vi "Create quad.vi"(1 "V3":sgl[](array[numeric]), 2 "V2":sgl[](array[numeric]), 3 "V1":sgl[](array[numeric]), 4 "V0":sgl[](array[numeric])) -> (0 "Quad":T1)   [LabVIEW 2014]
uses:
  Typedefs/Quad.ctl
  Dot product.vi
panel:
  # "PN 17/01/2015"
  # "Vertices"
  # "Edges"
  # "Unit normal"
  # "Edge unit normals"
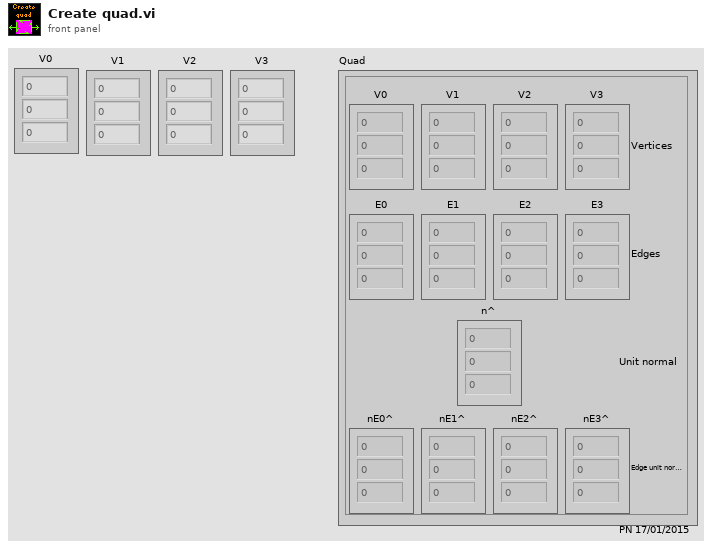
[diagram p1: front panel]
types:
  T1 = typedef "Quad.ctl" = cluster{"V0":sgl[], "V1":sgl[], "V2":sgl[], "V3":sgl[], "E0":sgl[], "E1":sgl[], "E2":sgl[], "E3":sgl[], "n^":sgl[], "nE0^":sgl[], "nE1^":sgl[], "nE2^":sgl[], "nE3^":sgl[]}
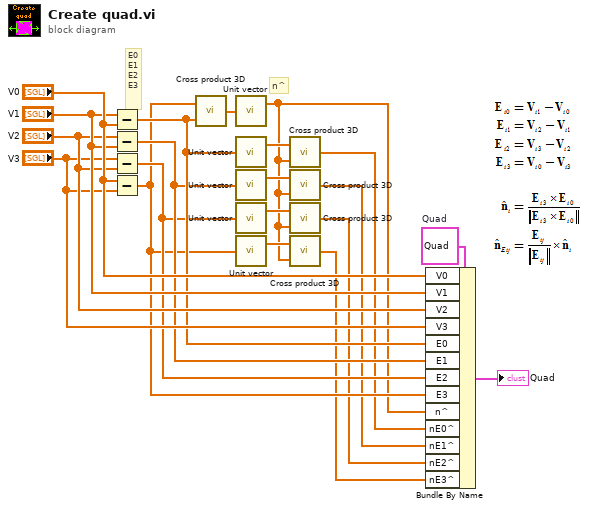
[diagram p0: block diagram]
diagram:
  w19 = T1 {"V0"=[], "V1"=[], "V2"=[], "V3"=[], "E0"=[], "E1"=[], "E2"=[], "E3"=[], "n^"=[], "nE0^"=[], "nE1^"=[], "nE2^"=[], "nE3^"=[]}  # Quad
  # "n^"
  # "E0\nE1\nE2\nE3"
  n1 = Subtract(x="V1", y="V0") -> (x-y=w10:sgl[])
  n2 = Subtract(x="V2", y="V1") -> (x-y=w9:sgl[])
  n3 = Subtract(x="V3", y="V2") -> (x-y=w8:sgl[])
  n4 = Subtract(x="V0", y="V3") -> (x-y=w7:sgl[])
  n5 = call "Cross product 3D.vi"("B"=w10, "A"=w7) -> ("A x B"=w20:sgl[])
  n6 = call "Unit vector.vi"("Vector"=w20) -> ("Unit vector"=w2:sgl[])  [unwired: 1 out]
  n7 = call "Unit vector.vi"("Vector"=w10) -> ("Unit vector"=w18:sgl[])  [unwired: 1 out]
  n8 = call "Unit vector.vi"("Vector"=w9) -> ("Unit vector"=w17:sgl[])  [unwired: 1 out]
  n9 = call "Unit vector.vi"("Vector"=w8) -> ("Unit vector"=w16:sgl[])  [unwired: 1 out]
  n10 = call "Unit vector.vi"("Vector"=w7) -> ("Unit vector"=w15:sgl[])  [unwired: 1 out]
  n11 = call "Cross product 3D.vi"("B"=w2, "A"=w18) -> ("A x B"=w6:sgl[])
  n12 = call "Cross product 3D.vi"("B"=w2, "A"=w17) -> ("A x B"=w5:sgl[])
  n13 = call "Cross product 3D.vi"("B"=w2, "A"=w16) -> ("A x B"=w4:sgl[])
  n14 = call "Cross product 3D.vi"("B"=w2, "A"=w15) -> ("A x B"=w3:sgl[])
  n15 = Bundle By Name(cluster=w19, "V0"="V0", "V1"="V1", "V2"="V2", "V3"="V3", "E0"=w10, "E1"=w9, "E2"=w8, "E3"=w7, "n^"=w2, "nE0^"=w6, "nE1^"=w5, "nE2^"=w4, "nE3^"=w3) -> (→"Quad":T1)
